vi "GetControlValueByPathArray.vi"(0 "VI Reference In":refnum<vi>, 5 "Control Path":string[](array[string]), 11 "error in":errorcluster) -> (4 "VI Reference Out":refnum<vi>, 6 "Value":variant, 15 "error out":errorcluster)   [LabVIEW 2016, in "Drona.lvlib" / "GetControlValue.lvlib"]
doc: "Gets the value of control which is specified.\n\nThe path of the control should be given in the successive index of the array"
uses:
  GetControlValue.lvlib
  GetControlRef/GetControlRef.lvlib
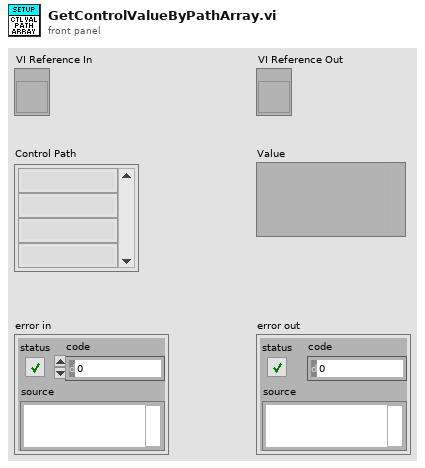
[diagram p1: front panel]
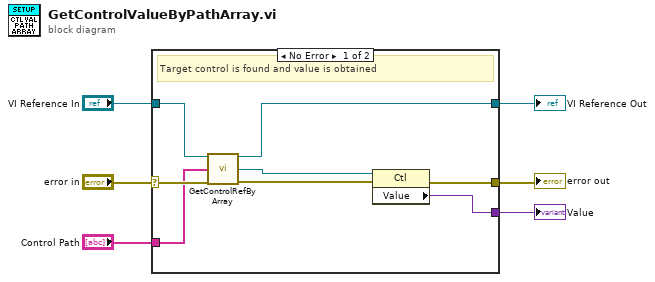
[diagram p0: block diagram]
diagram:
  n1 = case shown="No Error" "error in" {
    selector: "error in" -> [w12 w16]
    tunnel: "Control Path" -> [w9 _]
    tunnel: "VI Reference In" -> [w8 w15]
    tunnel: [w7 w15] -> w3
    tunnel: [w14 w16] -> w2
    tunnel: [w13 _] -> w1
    frame No Error {
      # "Target control is found and value is obtained"
      n2 = call "GetControlRefByArray.vi"("VI Reference In"=w8, "Control Path"=w9, "error In"=w12) -> ("VI Reference Out"=w7:refnum<vi>, "Ctl Refnum"=w10:refnum<vi>, "error out"=w11:errorcluster)  [unwired: 10 in]
      n3 = property class="Ctl"(reference=w10, error in=w11) -> (error out=w14:errorcluster, "Value"=w13:variant)  [unwired: 1 out]
    }
    frame Error {
    }
  }
  "error out" <- w2
  "VI Reference Out" <- w3
  "Value" <- w1
